vi "nufern_controller.vi"() -> ()   [LabVIEW 2014]
uses:
  <vilib>/FieldPoint/Polymorphic Read.llb/FP Read (Float Array).vi
  <vilib>/FieldPoint/Polymorphic Write.llb/FP Write (Float).vi
panel:
  in  "LEVEL CONTROL, 0-100 (%)":dbl(knob) scale=0.0..100.0
  in  "AMPLIFIER ENABLE":bool=TRUE
  out "Pre-amp Mon (Amps)":dbl format="%#_3g"
  out "Temp Mon (deg C)":dbl(slide) scale=0.0..100.0
  out "Mid Power Mon (Volts, no-cal)":dbl format="%#_3g"
  out "Out Power Mon (Volts, no-cal)":dbl format="%#_3g"
  out "+5 Vdc Out":dbl format="%#_3g"
  out "Power-Amp Pump Current (Amps)":dbl format="%#_3g"
  out "Seed Mon (Volts, no-cal)":dbl format="%#_3g"
  out "Back Refl. Mon (Volts, no-cal)":dbl format="%#_3g"
  out "Power Supply Fault":bool=TRUE
  out "Temp. Fault":bool=TRUE
  out "Back Refl. Fault":bool=TRUE
  out "Seed Power Fault":bool=TRUE
  out "Master Fault":bool=TRUE
  in  "Controller Stop":bool
  in  "Control Rate (ms)":u32=290
  # "FAULT STATUS"
  # "MONITORS"
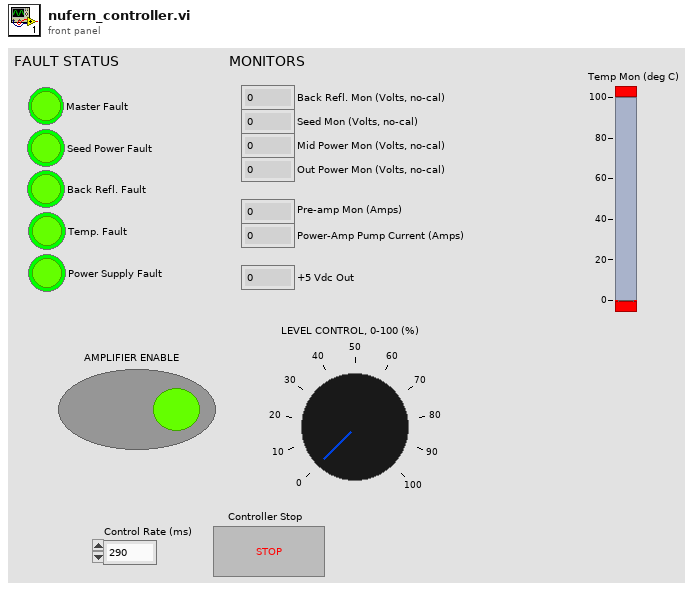
[diagram p1: front panel]
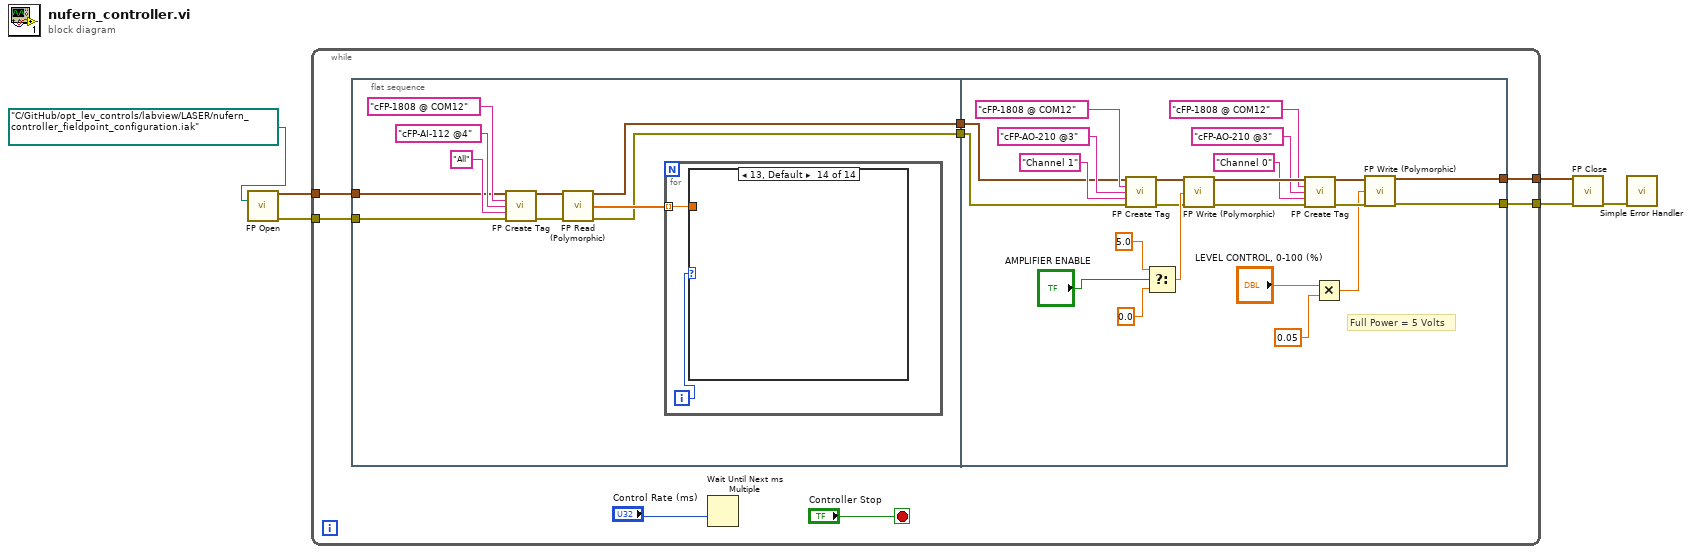
[diagram p0: block diagram]
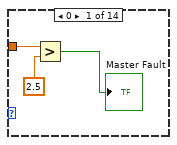
[diagram p2: hidden frame]
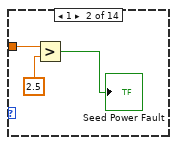
[diagram p3: hidden frame]
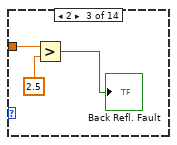
[diagram p4: hidden frame]
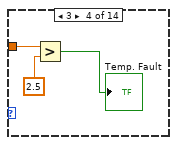
[diagram p5: hidden frame]
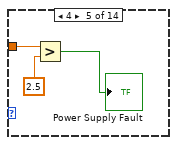
[diagram p6: hidden frame]
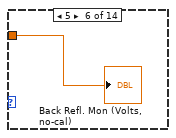
[diagram p7: hidden frame]
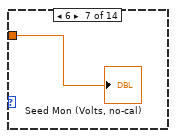
[diagram p8: hidden frame]
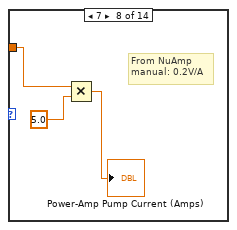
[diagram p9: hidden frame]
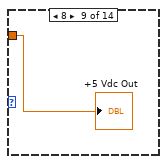
[diagram p10: hidden frame]
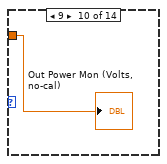
[diagram p11: hidden frame]
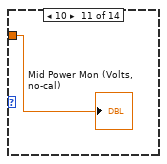
[diagram p12: hidden frame]
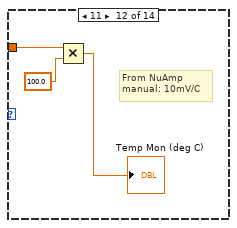
[diagram p13: hidden frame]
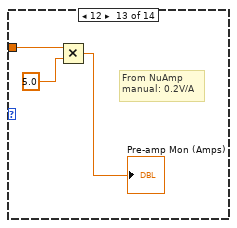
[diagram p14: hidden frame]
diagram:
  n1 = call <vilib>:"FP Open.vi"("iak file path"=path "C:/GitHub/opt_lev_controls/labview/LASER/nufern_controller_fieldpoint_configuration.iak") -> ("FP refnum out"=w6:cluster{"server refnum":u32, "tag refnum":u32}, "error out"=w5:errorcluster)  [unwired: 13 in]
  n2 = while {
    tunnel: w6 -> [w12]
    tunnel: w5 -> [w11]
    tunnel: [w8] -> w3
    tunnel: [w7] -> w2
    stop <- "Controller Stop" stop-if-true
    n3 = flat-sequence {
      tunnel: w12 -> [w18]
      tunnel: w11 -> [w17]
      tunnel: [w16] -> w10
      tunnel: [w15] -> w9
      tunnel: w10 -> [w75]
      tunnel: w9 -> [w74]
      tunnel: [w60] -> w8
      tunnel: [w59] -> w7
      frame #0 {
        n4 = call <vilib>:"FP Create Tag.vi"("FP refnum in"=w18, "comm resource name"="cFP-1808 @ COM12" ("Comm Resource Name"), "device name"="cFP-AI-112 @4" ("Device Name"), "item name"="All" ("Item Name"), "error in (no error)"=w17) -> ("FP refnum out"=w20:cluster{"server refnum":u32, "tag refnum":u32}, "error out"=w19:errorcluster)  [unwired: 9 in]
        n5 = call-poly <vilib>:"FP Read (Polymorphic).vi"("FP refnum in"=w20, "error in (no error)"=w19) -> ("FP refnum out"=w16:cluster{"server refnum":u32, "tag refnum":u32}, "values"=w24:dbl[], "error out"=w15:errorcluster)  [unwired: 10 in, 1 out]
        n6 = for {
          tunnel: w24 -> [w26] mode=indexing
          i -> [w25]
          n7 = case shown="13, Default" w25 {
            tunnel: w26 -> [w29 w32 w35 w38 w41 w42 w43 w46 w47 w48 w49 w51 w54 _]
            frame 0 {
              n8 = Greater?(x=w29, y=2.5) -> (0:→"Master Fault":bool)
            }
            frame 1 {
              n9 = Greater?(x=w32, y=2.5) -> (0:→"Seed Power Fault":bool)
            }
            frame 2 {
              n10 = Greater?(x=w35, y=2.5) -> (0:→"Back Refl. Fault":bool)
            }
            frame 3 {
              n11 = Greater?(x=w38, y=2.5) -> (0:→"Temp. Fault":bool)
            }
            frame 4 {
              n12 = Greater?(x=w41, y=2.5) -> (0:→"Power Supply Fault":bool)
            }
            frame 5 {
              "Back Refl. Mon (Volts, no-cal)" <- w42
            }
            frame 6 {
              "Seed Mon (Volts, no-cal)" <- w43
            }
            frame 7 {
              # "From NuAmp \nmanual: 0.2V/A"
              n13 = Multiply(x=w46, y=5.0) -> (x*y=→"Power-Amp Pump Current (Amps)":dbl)
            }
            frame 8 {
              "+5 Vdc Out" <- w47
            }
            frame 9 {
              "Out Power Mon (Volts, no-cal)" <- w48
            }
            frame 10 {
              "Mid Power Mon (Volts, no-cal)" <- w49
            }
            frame 11 {
              # "From NuAmp \nmanual: 10mV/C"
              n14 = Multiply(x=w51, y=100.0) -> (x*y=→"Temp Mon (deg C)":dbl)
            }
            frame 12 {
              # "From NuAmp \nmanual: 0.2V/A"
              n15 = Multiply(x=w54, y=5.0) -> (x*y=→"Pre-amp Mon (Amps)":dbl)
            }
            frame 13, Default {
            }
          }
        }
      }
      frame #1 {
        # "Full Power = 5 Volts"
        n16 = call <vilib>:"FP Create Tag.vi"("FP refnum in"=w75, "comm resource name"="cFP-1808 @ COM12" ("Comm Resource Name"), "device name"="cFP-AO-210 @3" ("Device Name"), "item name"="Channel 1" ("Item Name"), "error in (no error)"=w74) -> ("FP refnum out"=w69:cluster{"server refnum":u32, "tag refnum":u32}, "error out"=w68:errorcluster)  [unwired: 9 in]
        n17 = Select(t=5.0, s="AMPLIFIER ENABLE", f=0.0) -> (s? t:f=w70:dbl)
        n18 = call-poly <vilib>:"FP Write (Polymorphic).vi"("FP refnum in"=w69, "value"=w70, "error in (no error)"=w68) -> ("FP refnum out"=w67:cluster{"server refnum":u32, "tag refnum":u32}, "error out"=w66:errorcluster)  [unwired: 10 in, 1 out]
        n19 = call <vilib>:"FP Create Tag.vi"("FP refnum in"=w67, "comm resource name"="cFP-1808 @ COM12" ("Comm Resource Name"), "device name"="cFP-AO-210 @3" ("Device Name"), "item name"="Channel 0" ("Item Name"), "error in (no error)"=w66) -> ("FP refnum out"=w62:cluster{"server refnum":u32, "tag refnum":u32}, "error out"=w61:errorcluster)  [unwired: 9 in]
        n20 = Multiply(x="LEVEL CONTROL, 0-100 (%)", y=0.05) -> (x*y=w56:dbl)
        n21 = call-poly <vilib>:"FP Write (Polymorphic).vi"("FP refnum in"=w62, "value"=w56, "error in (no error)"=w61) -> ("FP refnum out"=w60:cluster{"server refnum":u32, "tag refnum":u32}, "error out"=w59:errorcluster)  [unwired: 10 in, 1 out]
      }
    }
    n22 = Wait Until Next ms Multiple(millisecond multiple="Control Rate (ms)") -> ()  [unwired: 1 out]
  }
  n23 = call <vilib>:"FP Close.vi"("FP refnum in"=w3, "error in (no error)"=w2) -> ("error out"=w4:errorcluster)  [unwired: 13 in]
  n24 = call <vilib>:"Simple Error Handler.vi"("error in (no error)"=w4) -> ()  [unwired: 4 in, 5 out]
